vi "Test Insert Row.vi"(11 "Test Case In":refnum<class "Test Open Xml.lvclass">) -> (0 "error out":errorcluster, 3 "Test Case Out":refnum<class "Test Open Xml.lvclass">)   [LabVIEW 2021, in "Test Open Xml.lvclass"]
uses:
  Test Open Xml.lvclass
  Test Open Xml.lvclass/Test Open Xml.ctl
  Source/Open Xml.lvlib
  <vilib>/Astemes/LUnit/Test Case.lvclass
  2ff6e858-e9c6-4c76-b040-d5cbb83ae7d3.vi
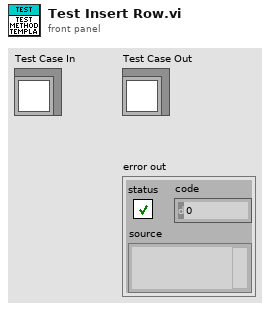
[diagram p1: front panel]
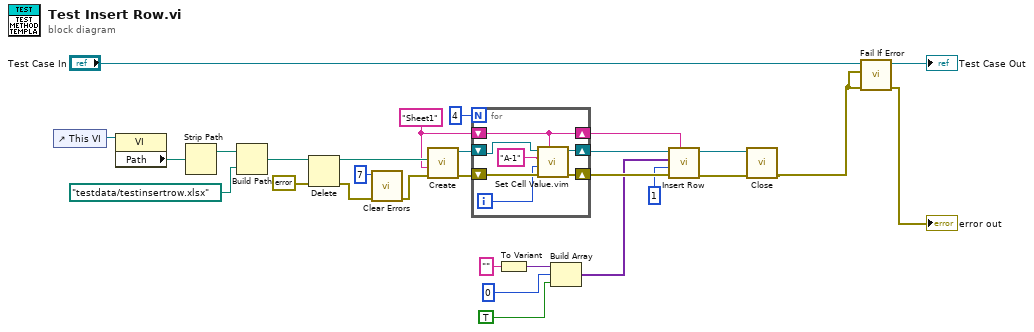
[diagram p0: block diagram]
diagram:
  w11 = "Sheet1" ("SheetName")
  n1 = control-ref of="This VI"() -> (w26:refnum<vi>)
  n2 = property class="VI"(reference=w26) -> ("Path"=w25:path)  [unwired: 1 in, 2 out]
  n3 = Strip Path(path=w25) -> (stripped path=w24:path)  [unwired: 1 out]
  n4 = Build Path(base path=w24, name or relative path=path "testdata/testinsertrow.xlsx") -> (appended path=w21:path)
  n5 = Delete(path (use dialog)=w21, error in=errorcluster {"status"=FALSE, "code"=0, "source"=""}) -> (deleted path=w20:path, error out=w22:errorcluster)  [unwired: 3 in, 1 out]
  n6 = call <vilib>:"Clear Errors.vi"("error in (no error)"=w22, "specific error code to clear (0: all)"=7) -> ("error out"=w19:errorcluster)  [unwired: 4 in, 1 out]
  n7 = call "Create.vi"("error in"=w19, "SheetName"=w11, "Path"=w20) -> ("error out"=w13:errorcluster, "SpreadsheetDocument"=w12:refnum<k24>)  [unwired: 7 in]
  n8 = for {
    N: 4 -> [_]
    shift-right: [w35] -> w10
    shift-left: w13 -> [w36]
    shift-right: [w32] -> w8
    shift-left: w12 -> [w33]
    shift-right: [w31] -> w7
    shift-left: w11 -> [w31]
    i -> [w30]
    n9 = call "Set Cell Value.vim"("Sheet Name"=w31, "error in"=w36, "Value"=w30, "Cell Address"="A-1", "SpreadsheetDoc in"=w33) -> ("error out"=w35:errorcluster, "SpreadsheetDoc out"=w32:refnum<k24>)  [unwired: 5 in]
  }
  n10 = To Variant(anything="") -> (Variant=w4:variant)
  n11 = Build Array(w4, 0, TRUE) -> (w1:variant[])
  n12 = call "Insert Row.vi"("SheetName"=w7, "error in"=w10, "Row Index"=1, "New Row"=w1, "SpreadsheetDocument in"=w8) -> ("error out"=w17:errorcluster, "SpreadsheetDocument out"=w16:refnum<k24>)  [unwired: 5 in]
  n13 = call "Close.vi"("error in"=w17, "SpreadsheetDocument"=w16) -> ("error out"=w15:errorcluster)  [unwired: 9 in]
  n14 = call <vilib>:"Fail If Error.vi"("error in (no error)"=w15, "Assert error"=w15, "LUnit Test Case In"="Test Case In") -> ("error out"=→"error out":errorcluster, "LUnit Test Case Out"=→"Test Case Out":refnum<class "Test Open Xml.lvclass">)  [unwired: 7 in]
